vi "Intake Cargo Call.vi"(3 "Right Button Values":bool[](array[boolean])) -> ()   [LabVIEW 2018]
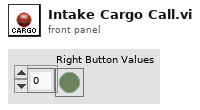
[diagram p1: front panel]
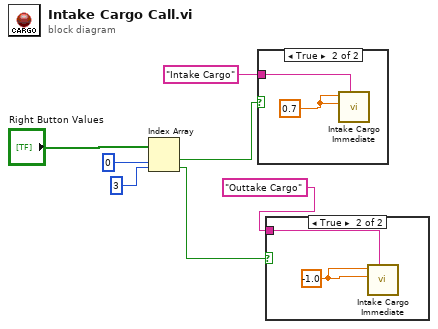
[diagram p0: block diagram]
diagram:
  n1 = Index Array(array="Right Button Values", index #1=0 ("index"), index #2=3 ("index")) -> (element #1=w5:bool, element #2=w1:bool)
  n2 = case shown="True" w5 {
    tunnel: "Intake Cargo" ("Description") -> [_ w8]
    frame False {
    }
    frame True {
      w9 = 0.7 ("Bottom Motor")
      n3 = call "Intake Cargo Immediate.vi"("Description"=w8, "Bottom Motor"=w9, "Top Motor"=w9) -> ()  [unwired: 8 in, 1 out]
    }
  }
  n4 = case shown="True" w1 {
    tunnel: "Outtake Cargo" ("Description") -> [_ w11]
    frame False {
    }
    frame True {
      w10 = -1.0 ("Bottom Motor")
      n5 = call "Intake Cargo Immediate.vi"("Description"=w11, "Bottom Motor"=w10, "Top Motor"=w10) -> ()  [unwired: 8 in, 1 out]
    }
  }
